vi "Update new NOK tests.vi"(11 "New NOK tests from previous DUT":string[](array[string])) -> (0 "error out":errorcluster)   [LabVIEW 2023, in "In a row NOK.lvlib"]
uses:
  In a row NOK.lvlib
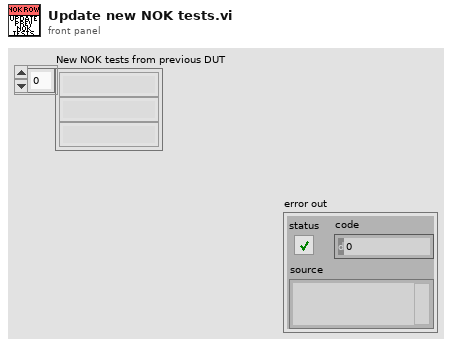
[diagram p1: front panel]
types:
  T1 = enum16{"open", "replace", "create", "open or create", "replace or create", "replace or create with confirmation"}
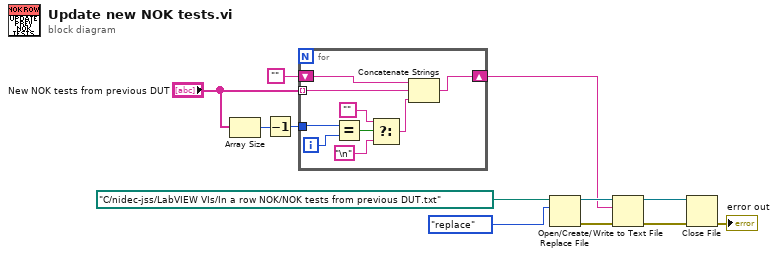
[diagram p0: block diagram]
diagram:
  n1 = Array Size(array="New NOK tests from previous DUT") -> (size(s)=w4:i32)
  n2 = Decrement(x=w4) -> (x-1=w3:i32)
  n3 = for {
    tunnel: "New NOK tests from previous DUT" -> [w21] mode=indexing
    shift-right: [w20] -> w2
    shift-left: "" -> [w19]
    tunnel: w3 -> [w18]
    i -> [w17]
    n4 = Equal?(x=w18, y=w17) -> (x = y?=w16:bool)
    n5 = Select(t="", s=w16, f="\n") -> (s? t:f=w13:string)
    n6 = Concatenate Strings(w19, w21, w13) -> (w20:string)
  }
  n7 = Open/Create/Replace File(file path (use dialog)=path "C:/nidec-jss/LabVIEW VIs/In a row NOK/NOK tests from previous DUT.txt", operation (0:open)=T1."replace") -> (refnum out=w11:refnum<file>, error out=w10:errorcluster)  [unwired: 4 in, 1 out]
  n8 = Write to Text File(file (use dialog)=w11, text=w2, error in=w10) -> (refnum out=w9:refnum<file>, error out=w8:errorcluster)  [unwired: 1 in, 1 out]
  n9 = Close File(refnum=w9, error in=w8) -> (error out=→"error out":errorcluster)  [unwired: 1 out]
